vi "Close Device Core.vi"(8 "error in (no error)":errorcluster, 11 "BNT_DAQmx-MCSV in":refnum<class "BNT_DAQmx-MCSV.lvclass">) -> (0 "error out":errorcluster, 3 "BNT_DAQmx-MCSV out":refnum<class "BNT_DAQmx-MCSV.lvclass">)   [LabVIEW 2016, in "BNT_DAQmx.lvlib" / "BNT_DAQmx-MCSV.lvclass"]
doc: "Close device driver connection."
uses:
  BNT_DAQmx-MCSV.lvclass
  BNT_DAQmx-MCSV.lvclass/BNT_DAQmx-MCSV.ctl
  CSPP_Core/Actors/CS++DeviceActor/CS++DeviceActor.lvclass
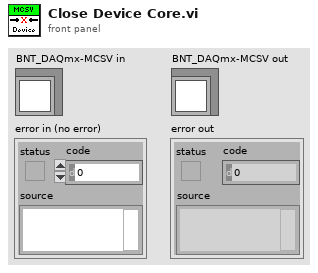
[diagram p1: front panel]
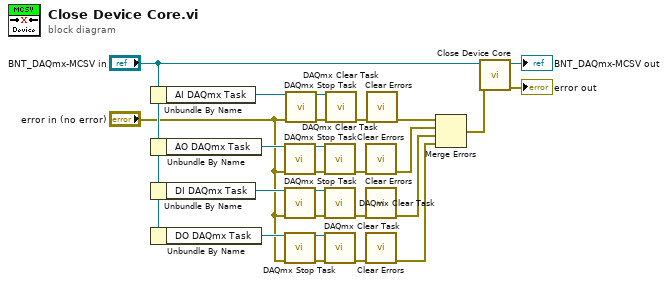
[diagram p0: block diagram]
diagram:
  n1 = Unbundle By Name("BNT_DAQmx-MCSV in") -> ("AI DAQmx Task"=w22:refnum<k21>)
  n2 = Unbundle By Name("BNT_DAQmx-MCSV in") -> ("AO DAQmx Task"=w17:refnum<k21>)
  n3 = Unbundle By Name("BNT_DAQmx-MCSV in") -> ("DI DAQmx Task"=w10:refnum<k21>)
  n4 = Unbundle By Name("BNT_DAQmx-MCSV in") -> ("DO DAQmx Task"=w7:refnum<k21>)
  n5 = call <vilib>:"DAQmx Stop Task.vi"("task/channels in"=w17, "error in"="error in (no error)") -> ("task out"=w13:refnum<k21>, "error out"=w16:errorcluster)  [unwired: 12 in]
  n6 = call <vilib>:"DAQmx Stop Task.vi"("task/channels in"=w10, "error in"="error in (no error)") -> ("task out"=w12:refnum<k21>, "error out"=w11:errorcluster)  [unwired: 12 in]
  n7 = call <vilib>:"DAQmx Stop Task.vi"("task/channels in"=w7, "error in"="error in (no error)") -> ("task out"=w5:refnum<k21>, "error out"=w6:errorcluster)  [unwired: 12 in]
  n8 = call <vilib>:"DAQmx Stop Task.vi"("task/channels in"=w22, "error in"="error in (no error)") -> ("task out"=w21:refnum<k21>, "error out"=w23:errorcluster)  [unwired: 12 in]
  n9 = call <vilib>:"DAQmx Clear Task.vi"("task in"=w13, "error in"=w16) -> ("error out"=w18:errorcluster)  [unwired: 13 in]
  n10 = call <vilib>:"DAQmx Clear Task.vi"("task in"=w12, "error in"=w11) -> ("error out"=w9:errorcluster)  [unwired: 13 in]
  n11 = call <vilib>:"DAQmx Clear Task.vi"("task in"=w5, "error in"=w6) -> ("error out"=w8:errorcluster)  [unwired: 13 in]
  n12 = call <vilib>:"DAQmx Clear Task.vi"("task in"=w21, "error in"=w23) -> ("error out"=w20:errorcluster)  [unwired: 13 in]
  n13 = call <vilib>:"Clear Errors.vi"("error in (no error)"=w18) -> ("error out"=w14:errorcluster)  [unwired: 5 in, 1 out]
  n14 = call <vilib>:"Clear Errors.vi"("error in (no error)"=w9) -> ("error out"=w2:errorcluster)  [unwired: 5 in, 1 out]
  n15 = call <vilib>:"Clear Errors.vi"("error in (no error)"=w8) -> ("error out"=w1:errorcluster)  [unwired: 5 in, 1 out]
  n16 = call <vilib>:"Clear Errors.vi"("error in (no error)"=w20) -> ("error out"=w19:errorcluster)  [unwired: 5 in, 1 out]
  n17 = Merge Errors(w19, w14, w2, w1) -> (w15:errorcluster)
  n18 = call-parent "Close Device Core.vi"("error in (no error)"=w15, "CS++DeviceActor in"="BNT_DAQmx-MCSV in") -> ("error out"=→"error out":errorcluster, "CS++DeviceActor out"=→"BNT_DAQmx-MCSV out":refnum<class "BNT_DAQmx-MCSV.lvclass">)  [unwired: 8 in]
